vi "SetLimits.vi"(8 "error in (no error)":errorcluster, 11 "DelayLineEmulate in":refnum<class "DLEmulate.lvclass">) -> (0 "error out":errorcluster, 3 "DelayLineEmulate out":refnum<class "DLEmulate.lvclass">)   [LabVIEW 2018, in "DLEmulate.lvclass"]
uses:
  DLEmulate.lvclass
  C:/Users/Sergey Denisov/Documents/REPS/TRANCON/Classes/GeneralFunctionality/GeneralFunctionality.lvclass
  DelayLineLS4/LS4_parameters.ctl
  GeneralFunctionality/GeneralFunctionality.lvclass/GeneralFunctionality.ctl
  Config/Config.lvclass
  DelayLine.lvclass
  GeneralFunctionality/GeneralFunctionality.lvclass
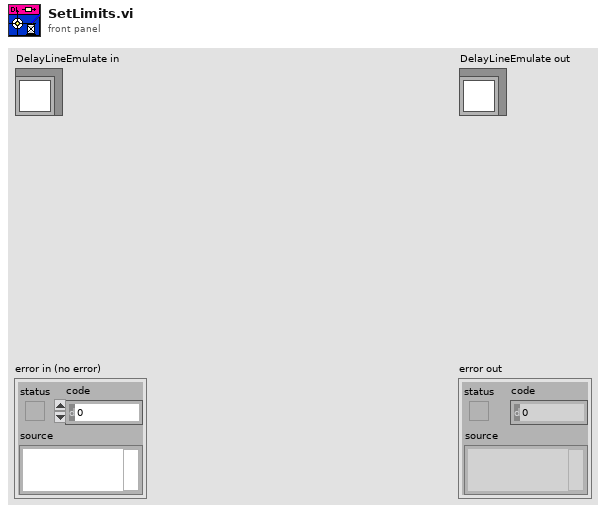
[diagram p1: front panel]
types:
  T1 = typedef "DelayLine.lvclass/LS4_parameters.ctl" = string
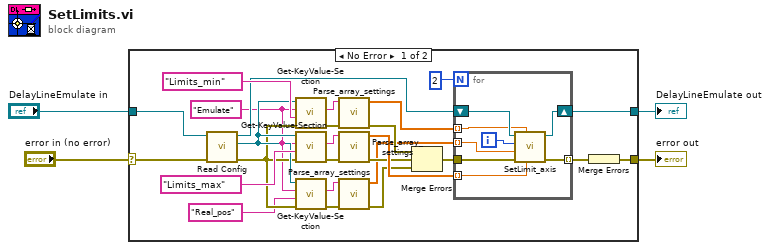
[diagram p0: block diagram]
diagram:
  n1 = case shown="No Error" "error in (no error)" {
    selector: "error in (no error)" -> [w18 w39]
    tunnel: [w6 w40] -> w2
    tunnel: "DelayLineEmulate in" -> [w19 w40]
    tunnel: [w5 w39] -> w1
    frame No Error {
      w9 = "Emulate" ("Section")
      n2 = call "Read Config.vi"("error in (no error)"=w18, "GeneralFunctionality en entrée"=w19) -> ("error out"=w10:errorcluster, "Config.lvclass"=w11:refnum<class "Config.lvclass">, "GeneralFunctionality en sortie"=w20:refnum<class "DLEmulate.lvclass">)  [unwired: 7 in]
      n3 = call-dynamic "Get-KeyValue-Section.vi"("error in (no error)"=w10, "Key"=T1 "Limits_min" ("Section"), "Section"=w9, "Config in"=w11) -> ("error out"=w29:errorcluster, "Value"=w30:string)  [unwired: 5 in, 1 out]
      n4 = call-dynamic "Get-KeyValue-Section.vi"("error in (no error)"=w10, "Key"=T1 "Limits_max" ("Section"), "Section"=w9, "Config in"=w11) -> ("error out"=w26:errorcluster, "Value"=w25:string)  [unwired: 5 in, 1 out]
      n5 = call-dynamic "Get-KeyValue-Section.vi"("error in (no error)"=w10, "Key"="Real_pos", "Section"=w9, "Config in"=w11) -> ("error out"=w14:errorcluster, "Value"=w7:string)  [unwired: 5 in, 1 out]
      n6 = call "Parse_array_settings.vi"("error in (no error)"=w29, "Value"=w30) -> ("error out"=w22:errorcluster, "Array"=w27:sgl[])  [unwired: 8 in]
      n7 = call "Parse_array_settings.vi"("error in (no error)"=w26, "Value"=w25) -> ("error out"=w21:errorcluster, "Array"=w23:sgl[])  [unwired: 8 in]
      n8 = call "Parse_array_settings.vi"("error in (no error)"=w14, "Value"=w7) -> ("error out"=w12:errorcluster, "Array"=w13:sgl[])  [unwired: 8 in]
      n9 = Merge Errors(w22, w21, w12) -> (w16:errorcluster)
      n10 = for {
        N: 2 -> [_]
        tunnel: w27 -> [w32] mode=indexing
        tunnel: w23 -> [w31] mode=indexing
        tunnel: [w36] -> w15 mode=indexing
        shift-right: [w37] -> w6
        shift-left: w20 -> [w38]
        tunnel: w16 -> [w35]
        tunnel: w13 -> [w33] mode=indexing
        i -> [w34]
        n11 = call-dynamic "SetLimit_axis.vi"("max"=w31, "min"=w32, "error in (no error)"=w35, "real pos zero"=w33, "Axis"=w34, "DelayLine in"=w38) -> ("error out"=w36:errorcluster, "DelayLine out"=w37:refnum<class "DLEmulate.lvclass">)  [unwired: 4 in]
      }
      n12 = Merge Errors(w15) -> (w5:errorcluster)
    }
    frame Error {
    }
  }
  "error out" <- w1
  "DelayLineEmulate out" <- w2
